vi "Close Global Event Log.vi"(8 "error in (no error)":errorcluster, 11 "Deferred Close Time (0 ms)":u32) -> (0 "error out":errorcluster)   [LabVIEW 2017, in "Singleton Event Log.lvlib"]
doc: "Close the global event log. If a deferred close time is defined, an asynchronous timer will be used to defer closing the log. Use this feature in a multi threaded applications where some modules may not be fully stopped when the close call occurs."
uses:
  <vilib>/gpm_packages/@cs/event-logger/Source/Composed Log/Singleton Event Log/Singleton Event Log.lvlib
  <vilib>/gpm_packages/@cs/event-logger/Source/Composed Log/LoggerReference/LoggerReference.lvclass
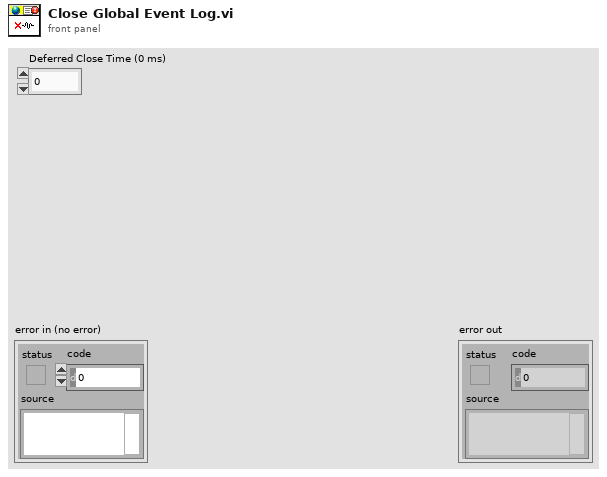
[diagram p1: front panel]
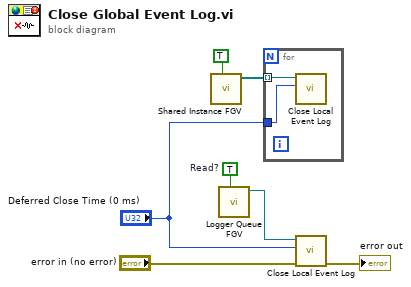
[diagram p0: block diagram]
diagram:
  w7 = TRUE  # Read?
  n1 = call <vilib>:"Shared Instance FGV.vi"("Read?"=TRUE) -> ("Shared Instances"=w2:refnum<class "LoggerReference.lvclass">[])  [unwired: 10 in]
  n2 = call <vilib>:"Logger Queue FGV.vi"("Read?"=w7) -> ("LogReference Instance Out"=w6:refnum<class "LoggerReference.lvclass">)  [unwired: 10 in]
  n3 = for {
    tunnel: w2 -> [w9] mode=indexing
    tunnel: "Deferred Close Time (0 ms)" -> [w8]
    n4 = call <vilib>:"Close Local Event Log.vi"("Deferred Close Time (0 ms)"=w8, "Log Instance"=w9) -> ()  [unwired: 9 in, 1 out]
  }
  n5 = call <vilib>:"Close Local Event Log.vi"("error in (no error)"="error in (no error)", "Deferred Close Time (0 ms)"="Deferred Close Time (0 ms)", "Log Instance"=w6) -> ("error out"=→"error out":errorcluster)  [unwired: 8 in]
